vi "Run by Point.vi"(4 "end Power":dbl, 6 "Power in":dbl, 8 "error in (no error)":errorcluster, 9 "y":dbl, 10 "x":dbl, 11 "RobotDriveDevRef":T1={"DevStatus"={"status"=FALSE, "code"=0, "source"=""}, "Motors[]"=[], "Square Inputs"=FALSE, "Max Output"=1.0}) -> (0 "error out":errorcluster, 1 "power out":dbl, 3 "refnum":T1={"DevStatus"={"status"=FALSE, "code"=0, "source"=""}, "Motors[]"=[], "Square Inputs"=FALSE, "Max Output"=1.0})   [LabVIEW 2017]
uses:
  <vilib>/Rock Robotics/WPI/RobotDrive/WPI_RobotDriveDevRef.ctl
  <vilib>/Rock Robotics/WPI/MotorControl/WPI_MotorControlDeviceRef.ctl
  <vilib>/Rock Robotics/WPI/MotorControl/WPI_MotorControlType.ctl
  <vilib>/Rock Robotics/SystemInterfaces/DIO/FPGA_DIOPWMChannel.ctl
  <vilib>/Rock Robotics/WPI/PWM/WPI_PWMDeadband.ctl
  <vilib>/Rock Robotics/SystemInterfaces/DIO/FPGA_DIOChannel.ctl
  Robot Global Data.vi
  <vilib>/Rock Robotics/WPI/RobotDrive/WPI_RobotDriveArcadeDrive_Standard(NoSaturation).vi
panel:
  out "y off":dbl
  out "x off":dbl
  out "distance left":dbl
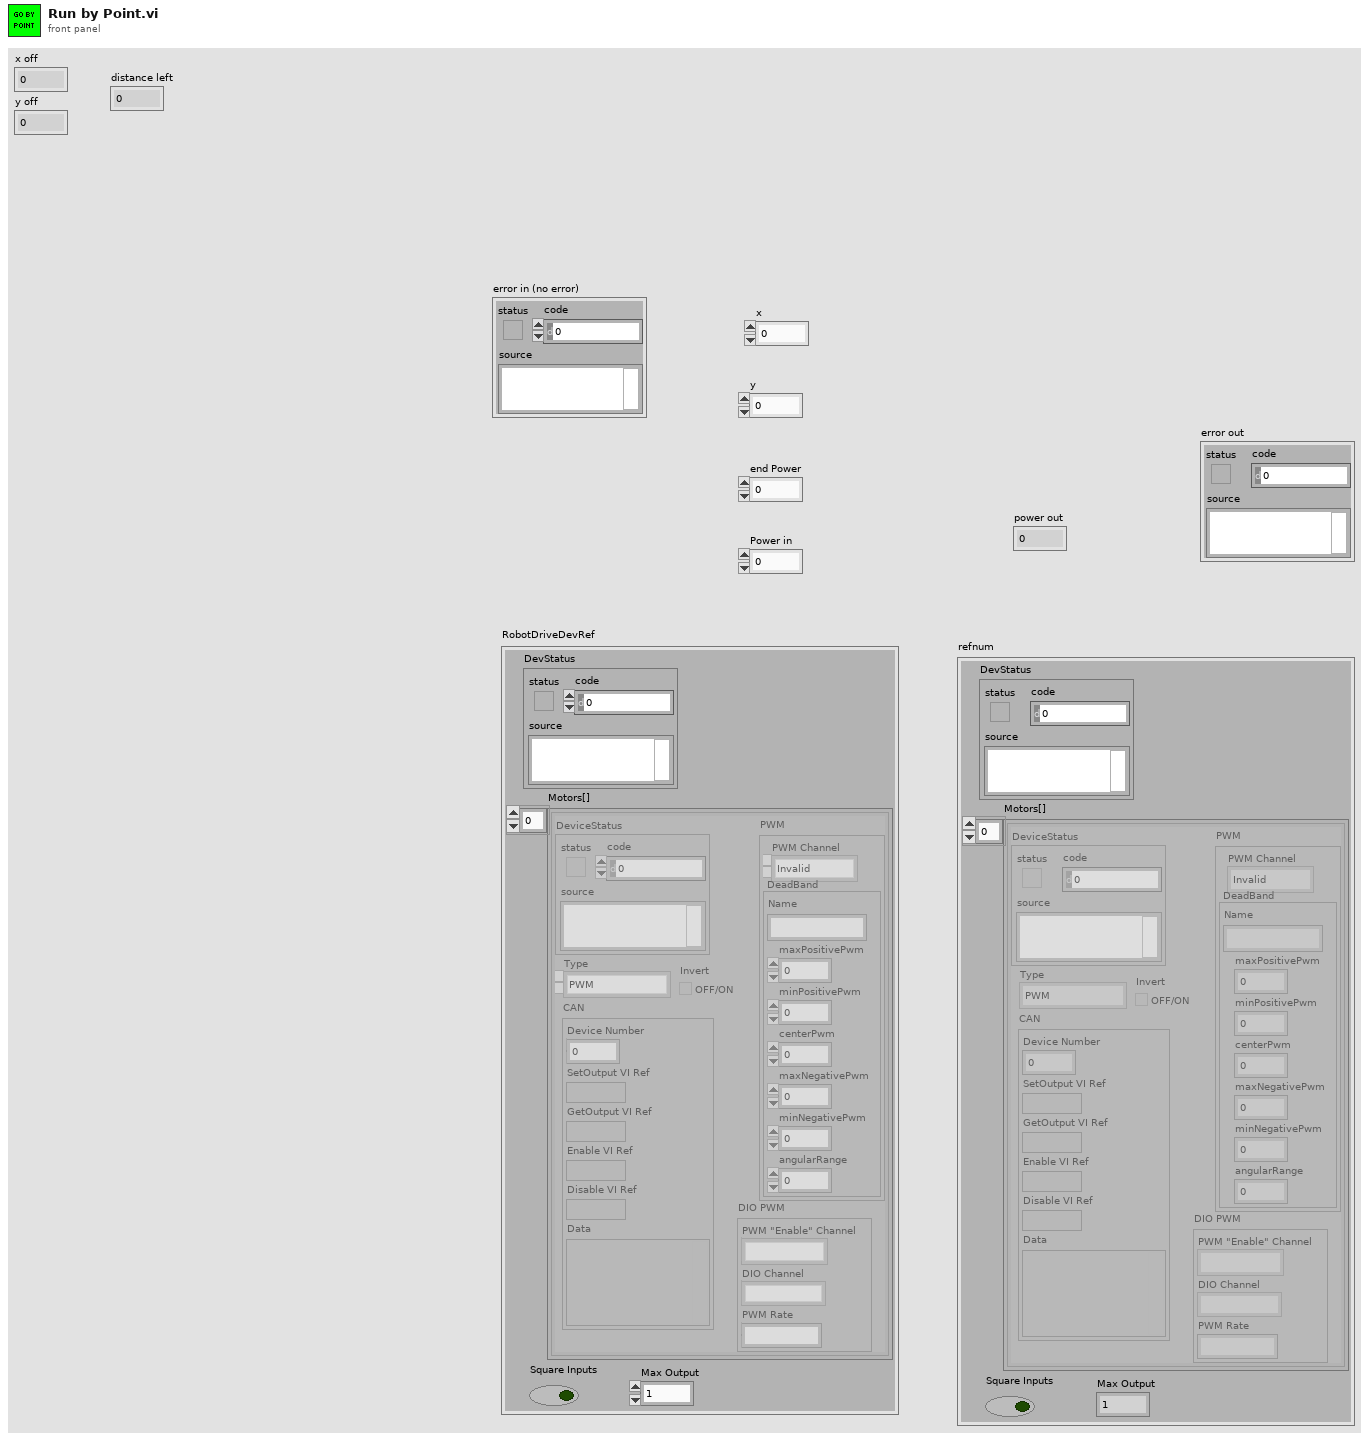
[diagram p1: front panel]
types:
  T1 = typedef "WPI_RobotDriveDevRef.ctl" = cluster{"DevStatus":errorcluster, "Motors[]":T2[], "Square Inputs":bool, "Max Output":dbl}
  T2 = typedef "WPI_MotorControlDeviceRef.ctl" = cluster{"DeviceStatus":errorcluster, "Type":T3, "PWM":cluster{"PWM Channel":T4, "DeadBand":T5}, "CAN":cluster{"Device Number":u8, "SetOutput VI Ref":variant, "GetOutput VI Ref":variant, "Enable VI Ref":variant, "Disable VI Ref":variant, "Data":variant}, "Invert":bool, "DIO PWM":cluster{"PWM \"Enable\" Channel":T4, "DIOChannel":T6, "PWM Rate":dbl}}
  T3 = typedef "WPI_MotorControlType.ctl" = enum16{"PWM", "CAN", "DIO PWM"}
  T4 = typedef "FPGA_DIOPWMChannel.ctl" = enum8{"PWM 0", "PWM 1", "PWM 2", "PWM 3", "PWM 4", "PWM 5", "PWM 6", "PWM 7", "PWM 8", "PWM 9", "PWM MXP 0", "PWM MXP 1", "PWM MXP 2", "PWM MXP 3", "PWM MXP 4", "PWM MXP 5", "PWM MXP 6", "PWM MXP 7", "PWM MXP 8", "PWM MXP 9", "Invalid"}
  T5 = typedef "WPI_PWMDeadband.ctl" = cluster{"Name":string, "maxPositivePwm":i32, "minPositivePwm":i32, "centerPwm":i32, "maxNegativePwm":i32, "minNegativePwm":i32, "angularRange":u16}
  T6 = typedef "FPGA_DIOChannel.ctl" = enum8{"DIO 0", "DIO 1", "DIO 2", "DIO 3", "DIO 4", "DIO 5", "DIO 6", "DIO 7", "DIO 8", "DIO 9", "DIO MXP 0", "DIO MXP 1", "DIO MXP 2", "DIO MXP 3", "DIO MXP 4", "DIO MXP 5", "DIO MXP 6", "DIO MXP 7", "DIO MXP 8", "DIO MXP 9", "DIO MXP 10", "DIO MXP 11", "DIO MXP 12", "DIO MXP 13", "DIO MXP 14", "DIO MXP 15", "SPI Port CS1", "SPI Port CS2", "SPI Port CS3", "SPI Port MISO", "SPI Port MOSI", "Invalid"}
  T7 = typedef "WPI_EncoderDevRef.ctl" = cluster{"DevStatus":errorcluster, "EncoderIndex":T8, "CounterIndex":T9, "DistancePerCount":dbl, "Decoding Type":T10}
  T8 = typedef "FPGA_EncoderIdx.ctl" = enum8{"Enc 0", "Enc 1", "Enc 2", "Enc 3", "Enc 4", "Enc 5", "Enc 6", "Enc 7", "Invalid"}
  T9 = typedef "FPGA_CounterCtrSystemIndex.ctl" = enum8{"Ctr 0", "Ctr 1", "Ctr 2", "Ctr 3", "Ctr 4", "Ctr 5", "Ctr 6", "Ctr 7", "Invalid"}
  T10 = typedef "WPI_EncoderType.ctl" = enum16{"1x", "2x", "4x"}
  T11 = cluster{"Yaw":dbl, "Roll":dbl, "Pitch":dbl, "Heading":dbl, "Fused Heading":dbl}
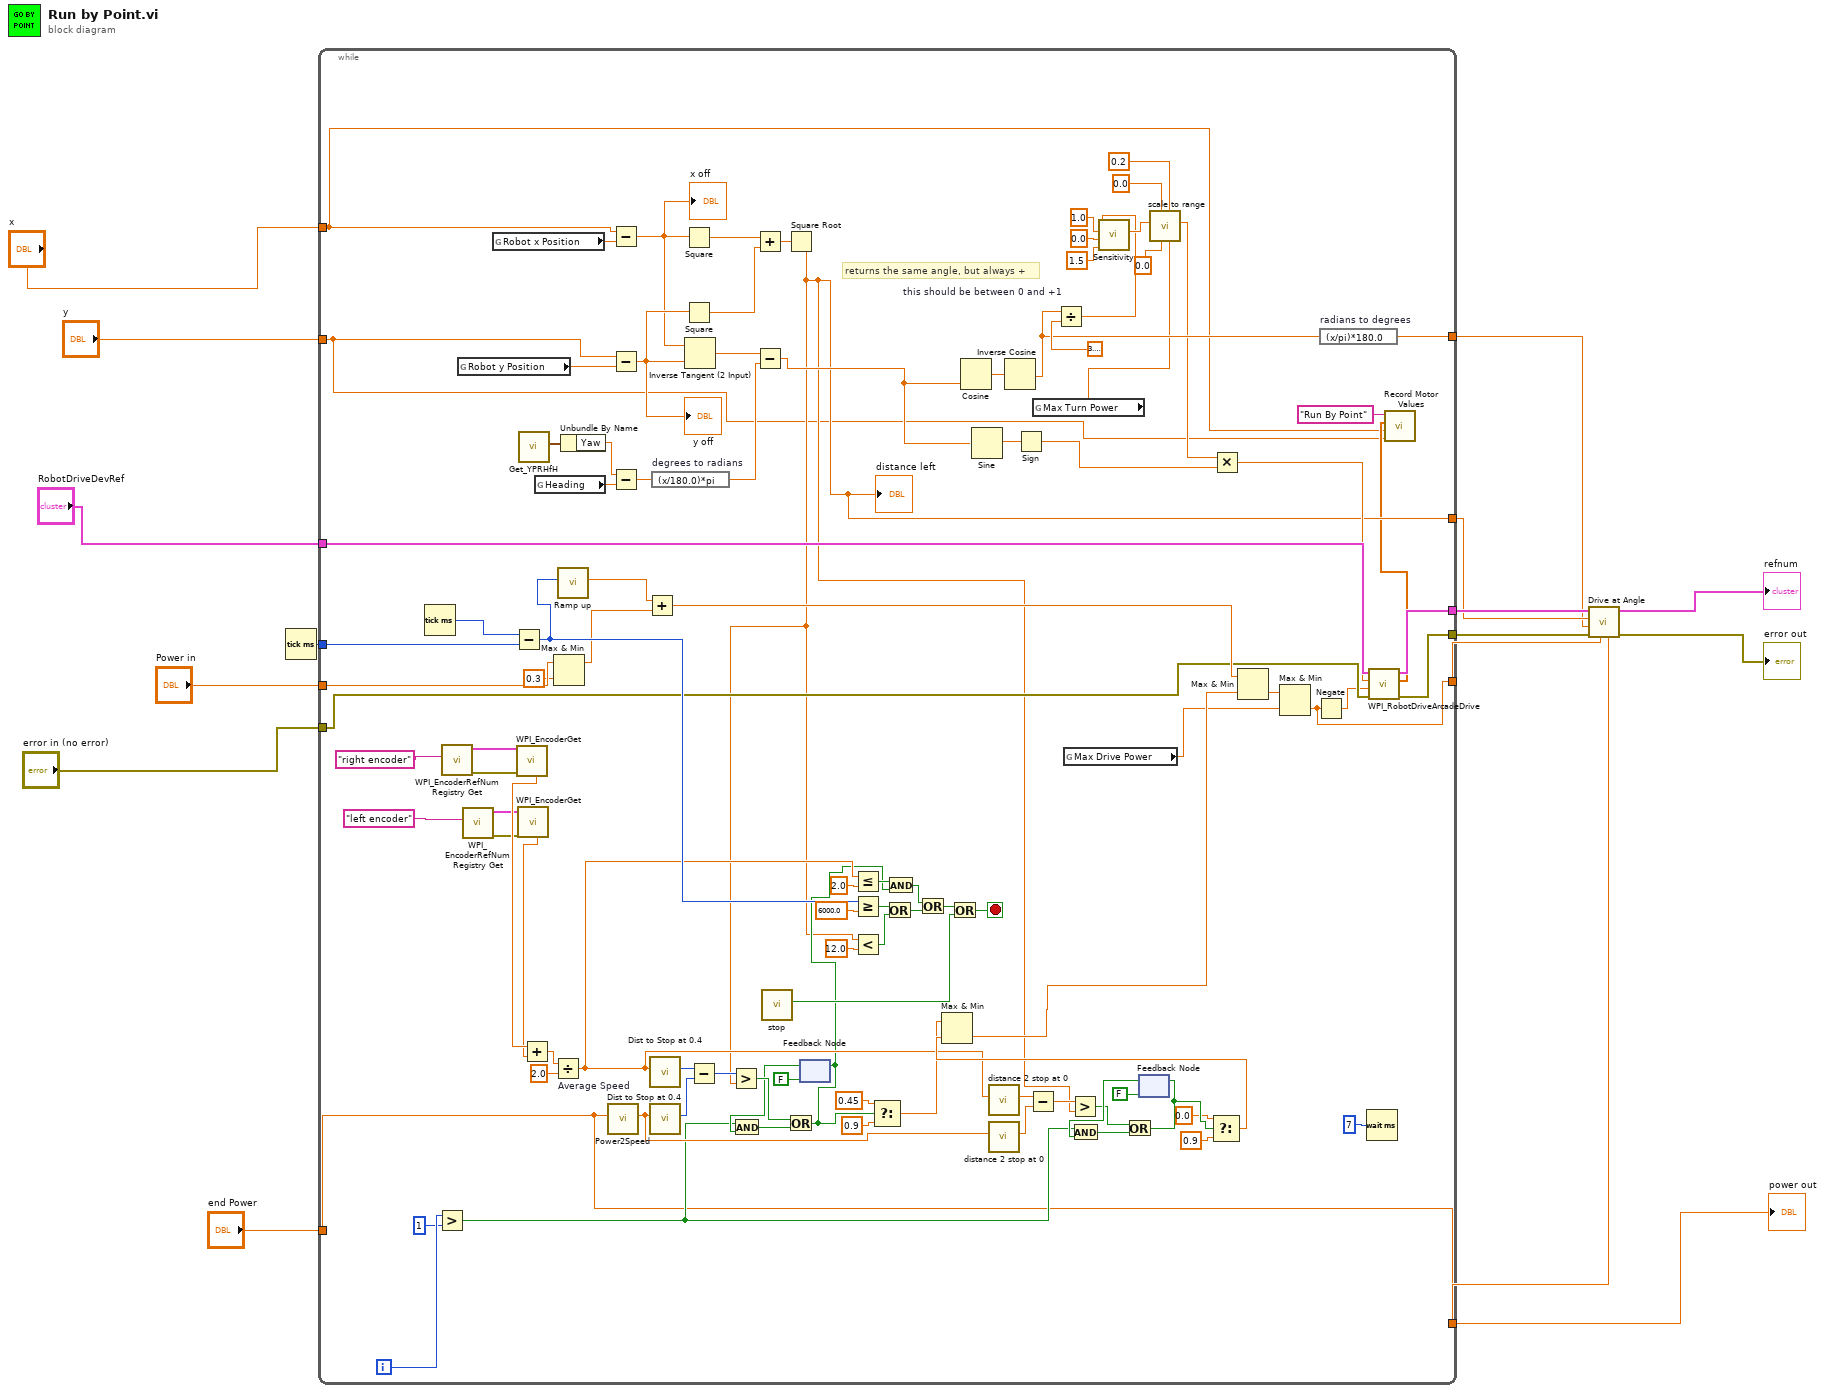
[diagram p0: block diagram]
diagram:
  n1 = Tick Count (ms)() -> (millisecond timer value=w15:u32)
  n2 = while {
    tunnel: [w118] -> w8
    tunnel: w15 -> [w48]
    tunnel: "error in (no error)" -> [w47]
    tunnel: "RobotDriveDevRef" -> [w46]
    tunnel: "end Power" -> [w36]
    tunnel: "Power in" -> [w23]
    tunnel: "x" -> [w25]
    tunnel: "y" -> [w24]
    tunnel: [w36] -> w1
    tunnel: [w33] -> w6
    tunnel: [w35] -> w7
    tunnel: [w34] -> w3
    tunnel: [w31] -> w2
    i -> [w74]
    stop <- w110 stop-if-true
    # "returns the same angle, but always +"
    n3 = Tick Count (ms)() -> (millisecond timer value=w116:u32)
    n4 = Greater?(x=w74, y=1) -> (0:w70:bool)
    n5 = call <vilib>:"WPI_EncoderRefNum Registry Get.vi"("refnum name"="right encoder") -> ("error out"=w44:errorcluster, "EncoderDevRef"=w45:T7)  [unwired: 9 in]
    n6 = global read "Robot Global Data.vi" "Robot y Position"() -> (w50:dbl)
    n7 = call <vilib>:"WPI_EncoderRefNum Registry Get.vi"("refnum name"="left encoder") -> ("error out"=w43:errorcluster, "EncoderDevRef"=w42:T7)  [unwired: 9 in]
    n8 = global read "Robot Global Data.vi" "Robot x Position"() -> (w51:dbl)
    n9 = Subtract(x=w116, y=w48) -> (x-y=w109:u32)
    n10 = call <vilib>:"WPI_EncoderGet.vi"("error in (no error)"=w44, "EncoderDevRef"=w45) -> ("Rate"=w103:dbl)  [unwired: 4 in, 5 out]
    n11 = call <vilib>:"WPI_EncoderGet.vi"("error in (no error)"=w43, "EncoderDevRef"=w42) -> ("Rate"=w102:dbl)  [unwired: 4 in, 5 out]
    n12 = call <vilib>:"Get_YPRHfH.vi"() -> ("YRPHfH"=w68:T11)  [unwired: 11 in]
    n13 = Add(x=w103, y=w102) -> (x+y=w104:dbl)
    n14 = global read "Robot Global Data.vi" "Heading"() -> (w64:dbl)
    n15 = Divide "Average Speed"(x=w104, y=2.0) -> (x/y=w77:dbl)
    n16 = Max & Min(x=w23, y=0.3) -> (max(x,y)=w21:dbl)  [unwired: 1 out]
    n17 = call "Ramp up.vi"("time"=w109) -> ("Power Out"=w108:dbl)  [unwired: 10 in]
    n18 = Unbundle By Name(w68) -> ("Yaw"=w65:dbl)
    n19 = call "Power2Speed.vi"("Power"=w36) -> ("Speed"=w91:dbl)  [unwired: 10 in]
    n20 = Subtract(x=w25, y=w51) -> (x-y=w52:dbl)
    "x off" <- w52
    n21 = Subtract(x=w24, y=w50) -> (x-y=w53:dbl)
    "y off" <- w53
    n22 = Subtract(x=w65, y=w64) -> (x-y=w54:dbl)
    n23 = Add(x=w108, y=w21) -> (x+y=w106:dbl)
    n24 = call "Dist to Stop at 0.4.vi"("Speed"=w77) -> ("Distance"=w101:i32)  [unwired: 10 in]
    n25 = call "Dist to Stop at 0.4.vi"("Speed"=w91) -> ("Distance"=w100:i32)  [unwired: 10 in]
    n26 = expression code="(x/180.0)*pi" "degrees to radians"(w54) -> (w55:dbl)
    n27 = Square(x=w52) -> (x^2=w57:dbl)
    n28 = Square(x=w53) -> (x^2=w58:dbl)
    n29 = Inverse Tangent (2 Input)(1:w53, 2:w52) -> (0:w69:dbl)
    n30 = Subtract(x=w101, y=w100) -> (x-y=w99:i32)
    n31 = Add(x=w57, y=w58) -> (x+y=w56:dbl)
    n32 = Subtract(x=w69, y=w55) -> (x-y=w49:dbl)
    n33 = call "stop.vi"() -> ("Boolean"=w112:bool)  [unwired: 11 in]
    n34 = Square Root(x=w56) -> (sqrt(x)=w34:dbl)
    "distance left" <- w34
    n35 = Greater?(x=w99, y=w34) -> (0:w98:bool)
    n36 = feedback #1(FALSE) -> (w97:bool)
    n37 = And(x=w70, y=w97) -> (x .and. y?=w72:bool)
    n38 = Or(x=w98, y=w72) -> (x .or. y?=w75:bool)
    n39 = feedback-in #1(w75) -> ()
    n40 = Less Or Equal?(x=w77, y=2.0) -> (x <= y?=w79:bool)
    n41 = Greater Or Equal?(x=w109, y=6000.0) -> (x >= y?=w114:bool)
    n42 = Less?(x=w34, y=12.0) -> (x < y?=w113:bool)
    n43 = Select(t=0.45, s=w75, f=0.9) -> (s? t:f=w82:dbl)
    n44 = Or(x=w114, y=w113) -> (x .or. y?=w111:bool)
    n45 = And(x=w79, y=w75) -> (x .and. y?=w76:bool)
    n46 = Or(x=w76, y=w111) -> (x .or. y?=w80:bool)
    n47 = Or(x=w80, y=w112) -> (x .or. y?=w110:bool)
    n48 = Cosine(x=w49) -> (cos(x)=w67:dbl)
    n49 = Sine(x=w49) -> (sin(x)=w66:dbl)
    n50 = call "distance 2 stop at 0.vi"("speed"=w77) -> ("Distance"=w93:dbl)  [unwired: 10 in]
    n51 = call "distance 2 stop at 0.vi"("speed"=w91) -> ("Distance"=w92:dbl)  [unwired: 10 in]
    n52 = Inverse Cosine(1:w67) -> (0:w30:dbl)
    n53 = Sign(1:w66) -> (0:w59:dbl)
    n54 = Subtract(x=w93, y=w92) -> (x-y=w90:dbl)
    n55 = global read "Robot Global Data.vi" "Max Turn Power"() -> (w29:dbl)
    n56 = Divide "this should be between 0 and +1"(x=w30, y=3.141592653589793) -> (x/y=w19:dbl)
    n57 = global read "Robot Global Data.vi" "Max Drive Power"() -> (w37:dbl)
    n58 = Greater?(x=w90, y=w34) -> (0:w84:bool)
    n59 = call "Sensitivity.vi"("Sensitivity"=1.5, "Low"=0.0, "High"=1.0, "Signal"=w19) -> ("Output"=w20:dbl)  [unwired: 7 in]
    n60 = feedback #2(FALSE) -> (w88:bool)
    n61 = And(x=w70, y=w88) -> (x .and. y?=w71:bool)
    n62 = Or(x=w84, y=w71) -> (x .or. y?=w89:bool)
    n63 = feedback-in #2(w89) -> ()
    n64 = call "scale to range.vi"("Max"=w29, "High"=0.2, "Min"=0.0, "Low"=0.0, "In Signal"=w20) -> ("Output signal"=w28:dbl)  [unwired: 6 in]
    n65 = Select(t=0.0, s=w89, f=0.9) -> (s? t:f=w83:dbl)
    n66 = Max & Min(x=w82, y=w83) -> (min(x,y)=w81:dbl)  [unwired: 1 out]
    n67 = Multiply(x=w28, y=w59) -> (x*y=w39:dbl)
    n68 = Max & Min(x=w106, y=w81) -> (min(x,y)=w107:dbl)  [unwired: 1 out]
    n69 = Max & Min(x=w107, y=w37) -> (min(x,y)=w33:dbl)  [unwired: 1 out]
    n70 = Negate(x=w33) -> (-x=w32:dbl)
    n71 = expression code="(x/pi)*180.0" "radians to degrees"(w30) -> (w31:dbl)
    n72 = Wait (ms)(milliseconds to wait=u32 7) -> ()  [unwired: 1 out]
    n73 = call-poly <vilib>:"WPI_RobotDriveArcadeDrive.vi"("error in (no error)"=w47, "Y axis value"=w32, "X axis value"=w39, "RobotDriveDevRef"=w46) -> ("error out"=w35:errorcluster, "Motor Values"=w26:dbl[], "RobotDriveDevRef"=w118:T1)  [unwired: 5 out]
    n74 = call "Record Motor Values.vi"("Target1 2"=w24, "Target1"=w25, "Motor Values"=w26, "VI Block Name"="Run By Point") -> ()  [unwired: 8 in]
  }
  "power out" <- w1
  n75 = call "Drive at Angle.vi"("end power"=w1, "Begin power"=w6, "error in (no error)"=w7, "Angle"=w2, "Distance"=w3, "RobotDriveDevRef"=w8) -> ("error out"=→"error out":errorcluster, "refnum"=→"refnum":T1)  [unwired: 3 in, 1 out]
